vi "Stop Sequence.vi"(8 "error in (no error)":errorcluster, 10 "Use previous step values for Last values":bool, 11 "Output Sequencer in":refnum<class "Output Sequencer.lvclass">) -> (0 "error out":errorcluster, 2 "Sequencer State":T1, 3 "Output Sequencer out":refnum<class "Output Sequencer.lvclass">)   [LabVIEW 2020, in "Output Sequencer.lvlib" / "Output Sequencer.lvclass"]
uses:
  Output Sequencer.lvclass
  Types/Sequencer State.ctl
  Output Sequencer.lvclass/Output Sequencer.ctl
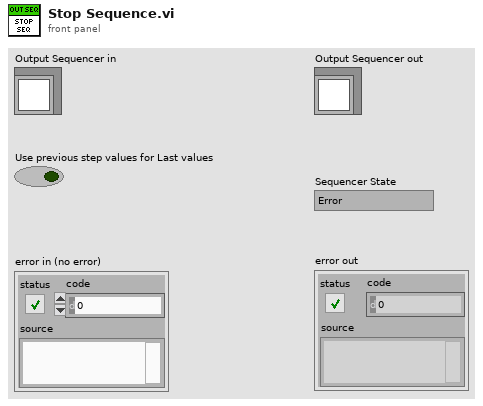
[diagram p1: front panel]
types:
  T1 = typedef "Output Sequencer.lvlib/Output Sequencer.lvclass/Sequencer State.ctl" = enum16{"Error", "Initialize", "Prepare channels", "Wait for test", "Wait for %.1f sec", "Wait for trigger", "Stop condition", "Wait for resume", "Running", "Paused", "No valid step", "Stopped"}
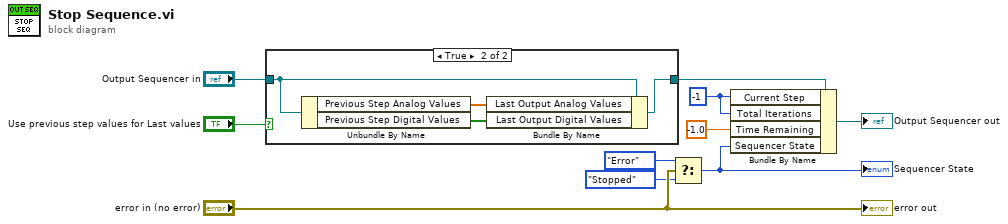
[diagram p0: block diagram]
diagram:
  w10 = -1 ("Current Sequence ID")
  n1 = case shown="True" "Use previous step values for Last values" {
    tunnel: "Output Sequencer in" -> [w11 w15]
    tunnel: [w11 w12] -> w5
    frame False {
    }
    frame True {
      n2 = Unbundle By Name(w15) -> ("Previous Step Analog Values"=w14:dbl[], "Previous Step Digital Values"=w13:bool[])
      n3 = Bundle By Name(cluster=w15, "Last Output Analog Values"=w14, "Last Output Digital Values"=w13) -> (w12:refnum<class "Output Sequencer.lvclass">)
    }
  }
  n4 = Select(t=Sequencer_State."Error" ("State.Sequencer State"), s="error in (no error)", f=Sequencer_State."Stopped" ("State.Sequencer State")) -> (s? t:f=w1:T1)
  "Sequencer State" <- w1
  n5 = Bundle By Name(cluster=w5, "Current Step"=w10, "Total Iterations"=w10, "Time Remaining"=-1.0, "Sequencer State"=w1) -> (→"Output Sequencer out":refnum<class "Output Sequencer.lvclass">)
  "error out" <- "error in (no error)"
